vi "Main.vi"() -> ()   [LabVIEW 2015]
doc: "The myRIO Project template acquires acceleration data from the onboard accelerometer and displays the changes of acceleration values in a waveform chart."
uses:
  <vilib>/myRIO/Instrument Drivers/Onboard IO/PWM/typedefs/PWM Reference.ctl
  <vilib>/myRIO/Common/Instrument Driver Framework/Utilities/typedefs/myRIO Generic Hardware Reference.ctl
  <vilib>/myRIO/Common/Instrument Driver Framework/Utilities/typedefs/Hardware Version Enum.ctl
  <vilib>/myRIO/Common/Instrument Driver Framework/Utilities/typedefs/myRIO v1.0 Reference.ctl
  <vilib>/myRIO/Common/Instrument Driver Framework/Utilities/typedefs/Generic FPGA Reference.ctl
  <vilib>/myRIO/Common/Instrument Driver Framework/myRIO v1.0/PWM/typedefs/PWM Channels Enum.ctl
  <vilib>/myRIO/Instrument Drivers/Onboard IO/PWM/typedefs/PWM Configuration.ctl
  <vilib>/userdefined/High Color/nirio_resource_hc.ctl
  <vilib>/myRIO/Instrument Drivers/Onboard IO/DIO/typedefs/DIO Reference.ctl
  <vilib>/myRIO/Common/Instrument Driver Framework/myRIO v1.0/DIO/typedefs/DIO Channels List.ctl
  <vilib>/myRIO/Common/Instrument Driver Framework/myRIO v1.0/DIO/typedefs/DIO Channels Enum.ctl
  <vilib>/myRIO/Instrument Drivers/Onboard Devices/Accelerometer/typedefs/Accelerometer Reference.ctl
  <vilib>/myRIO/Common/Instrument Driver Framework/myRIO v1.0/Accelerometer/typedefs/Accelerometer Channels List.ctl
  <vilib>/myRIO/Common/Instrument Driver Framework/myRIO v1.0/Accelerometer/typedefs/Accelerometer Channels Enum.ctl
  <vilib>/myRIO/Common/Instrument Driver Framework/Utilities/vis/Is FPGA Ref Available.vi
  <vilib>/myRIO/Common/Instrument Driver Framework/myRIO v1.0/DIO/vis/myRIO v1.1 Open DIO.vi
  <vilib>/myRIO/Instrument Drivers/Onboard IO/DIO/vis/Read.vi
  <vilib>/myRIO/Instrument Drivers/Onboard IO/DIO/vis/Write.vi
  <vilib>/myRIO/Common/Instrument Driver Framework/myRIO v1.0/PWM/vis/myRIO v1.1 Open PWM.vi
  <vilib>/myRIO/Instrument Drivers/Onboard IO/PWM/vis/Set Duty Cycle and Frequency.vi
  <vilib>/myRIO/Common/Instrument Driver Framework/myRIO v1.0/Accelerometer/vis/myRIO v1.1 Open Accelerometer.vi
  <vilib>/myRIO/Instrument Drivers/Onboard Devices/Accelerometer/vis/Read.vi
  <vilib>/myRIO/Common/Instrument Driver Framework/Utilities/vis/Validate Channels.vi
  <vilib>/myRIO/Common/Instrument Driver Framework/myRIO v1.0/DIO/vis/myRIO v1.0 Reserve DIO.vi
  <vilib>/myRIO/Common/Instrument Driver Framework/myRIO v1.0/PWM/vis/myRIO v1.0 Reserve PWM.vi
  <vilib>/myRIO/Common/Instrument Driver Framework/myRIO v1.0/Accelerometer/vis/myRIO v1.0 Reserve Accelerometer.vi
  <vilib>/myRIO/Common/Instrument Driver Framework/myRIO v1.0/UART/vis/myRIO v1.0 Close UART.vi
  <vilib>/myRIO/Common/Instrument Driver Framework/myRIO v1.0/Resource Manager/vis/myRIO v1.0 Reserve Channel List.vi
  <vilib>/myRIO/Common/Instrument Driver Framework/myRIO v1.0/DIO/vis/myRIO v1.0 Build MUX Configuration DIO.vi
  <vilib>/myRIO/Common/Instrument Driver Framework/myRIO v1.0/PWM/vis/myRIO v1.0 Build MUX Configuration PWM.vi
  <vilib>/myRIO/Common/Instrument Driver Framework/myRIO v1.0/Accelerometer/vis/myRIO v1.0 Build MUX Configuration Accelerometer.vi
  <vilib>/myRIO/Common/Instrument Driver Framework/myRIO v1.0/Resource Manager/vis/myRIO v1.0 Reserve Channel.vi
  <vilib>/myRIO/Common/Instrument Driver Framework/myRIO v1.0/Resource Manager/vis/myRIO v1.0 Unreserve Channel.vi
  <vilib>/myRIO/Common/Instrument Driver Framework/myRIO v1.0/Resource Manager/vis/myRIO v1.0 Create Configuration List.vi
  <vilib>/myRIO/Common/Instrument Driver Framework/myRIO v1.0/Resource Manager/vis/myRIO v1.0 Build Mutex Name.vi
  <vilib>/Utility/VariantDataType/GetNumericInfo.vi
  <vilib>/Utility/error.llb/Error Cluster From Error Code.vi
  <vilib>/myRIO/Common/Instrument Driver Framework/myRIO v1.0/myRIO v1.1 Open.vi
  <vilib>/myRIO/Common/Instrument Driver Framework/Utilities/vis/IO Manager.vi
  <vilib>/myRIO/Common/Instrument Driver Framework/Utilities/vis/Configuration Manager.vi
  <vilib>/myRIO/Common/Instrument Driver Framework/myRIO v1.0/Resource Manager/vis/myRIO v1.0 Configure IO.vi
  <vilib>/myRIO/Common/Instrument Driver Framework/myRIO v1.0/myRIO v1.0 Close.vi
  <vilib>/myRIO/Common/Instrument Driver Framework/myRIO v1.0/DIO/vis/myRIO v1.0 Write DIO.vi
  <vilib>/myRIO/Common/Instrument Driver Framework/myRIO v1.0/PWM/vis/myRIO v1.0 Write PWM.vi
  <vilib>/myRIO/Common/Instrument Driver Framework/myRIO v1.0/DIO/vis/myRIO v1.0 Read DIO.vi
  <vilib>/myRIO/Common/Instrument Driver Framework/myRIO v1.0/Accelerometer/vis/myRIO v1.0 Get Scaling Constant Accelerometer.vi
  <vilib>/myRIO/Common/Instrument Driver Framework/myRIO v1.0/Accelerometer/vis/myRIO v1.0 Read Accelerometer.vi
  <vilib>/myRIO/Common/Instrument Driver Framework/Utilities/vis/FPGA Ref Manager.vi
  <vilib>/myRIO/Common/Instrument Driver Framework/myRIO v1.0/myRIO v1.0 Reset FPGA.vi
  <vilib>/myRIO/Common/Instrument Driver Framework/myRIO v1.0/IRQ/vis/myRIO v1.0 IRQ Info FGV.vi
  <vilib>/myRIO/Common/Instrument Driver Framework/myRIO v1.0/IRQ/vis/myRIO v1.0 Timer IRQ Info FGV.vi
  <vilib>/myRIO/Common/Instrument Driver Framework/myRIO v1.0/IRQ/vis/myRIO v1.0 ISR Agent.vi
  <vilib>/myRIO/Express VI/Onboard IO/DO/DO Express VI.xnode
  <vilib>/myRIO/Instrument Drivers/Onboard IO/DIO/vis/myRIO DIO Open.xnode
  <vilib>/myRIO/Express VI/Onboard IO/PWM/PWM Express VI.xnode
  <vilib>/myRIO/Instrument Drivers/Onboard IO/PWM/vis/myRIO PWM Open.xnode
  <vilib>/myRIO/Express VI/Onboard IO/DI/DI Express VI.xnode
  <vilib>/myRIO/Express VI/Onboard Devices/Accelerometer/Accelerometer Express VI.xnode
  <vilib>/myRIO/Instrument Drivers/Onboard Devices/Accelerometer/vis/myRIO Accelerometer Open.xnode
  <vilib>/myRIO/Instrument Drivers/Utilities/Utilities.lvlib
  <vilib>/myRIO/Instrument Drivers/Onboard Devices/Accelerometer/Accelerometer.lvlib
  <vilib>/myRIO/Instrument Drivers/Onboard IO/PWM/PWM.lvlib
  <vilib>/myRIO/Instrument Drivers/Onboard IO/DIO/DIO.lvlib
  <vilib>/ptbypt/NI_PtbyPt.lvlib
panel:
  out "结果":dbl
  out "X-Axis":dbl
  out "波形图表":T1(graph)
  out "error out":errorcluster
  # "Overview: The myRIO Project template acquires acceleration data from the onboard accelerometer and displays the changes of acceleration values in a waveform chart.\nInstructions:\n1. Check the myRIO target IP address in the project and make sure the target IP address is correct. \n2. Run this VI."
  # "左 29"
  # "右31"
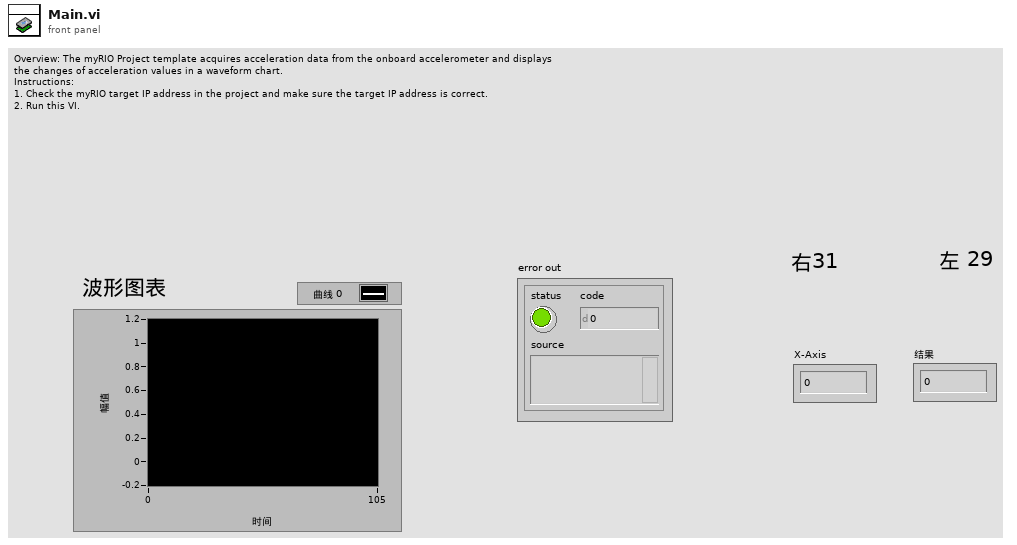
[diagram p1: front panel]
types:
  T1 = cluster{"X-Axis":dbl, "Y-Axis":dbl, "Z-Axis":dbl}
  T2 = typedef "PWM.lvlib/PWM Reference.ctl" = cluster{"myRIO Reference":T3, "PWM Channels Enum":T7, "PWM Configuration":T8}
  T3 = typedef "myRIO Generic Hardware Reference.ctl" = cluster{"myRIO Model":T4, "myRIO Hardware Reference":T5}
  T4 = typedef "Hardware Version Enum.ctl" = enum16{"Unknown", "myRIO-1900", "myRIO-1950", "roboRIO"}
  T5 = typedef "myRIO v1.0 Reference.ctl" = cluster{"Generic FPGA Reference":T6, "Allow multiple opens":bool}
  T6 = typedef "Generic FPGA Reference.ctl" = refnum<k20>
  T7 = typedef "PWM Channels Enum.ctl" = enum16{"Not Connected", "C/PWM0", "C/PWM1", "A/PWM0", "A/PWM1", "A/PWM2", "B/PWM0", "B/PWM1", "B/PWM2", "PWM/PWM0", "PWM/PWM1", "PWM/PWM2", "PWM/PWM3", "PWM/PWM4", "PWM/PWM5", "PWM/PWM6", "PWM/PWM7", "PWM/PWM8", "PWM/PWM9"}
  T8 = typedef "PWM.lvlib/PWM Configuration.ctl" = cluster{"Frequency":dbl, "Duty Cycle":dbl}
  T9 = typedef "nirio_resource_hc.ctl" = tag
  T10 = typedef "DIO.lvlib/DIO Reference.ctl" = cluster{"myRIO Reference":T3, "DIO Channels List":T11}
  T11 = typedef "DIO Channels List.ctl" = T12[]
  T12 = typedef "DIO Channels Enum.ctl" = enum16{"Not Connected", "C/DIO0", "C/DIO1", "C/DIO2", "C/DIO3", "C/DIO4", "C/DIO5", "C/DIO6", "C/DIO7", "A/DIO0", "A/DIO1", "A/DIO2", "A/DIO3", "A/DIO4", "A/DIO5", "A/DIO6", "A/DIO7", "A/DIO8", "A/DIO9", "A/DIO10", "A/DIO11", "A/DIO12", "A/DIO13", "A/DIO14", "A/DIO15", "B/DIO0", "B/DIO1", "B/DIO2", "B/DIO3", "B/DIO4", "B/DIO5", "B/DIO6", "B/DIO7", "B/DIO8", "B/DIO9", "B/DIO10", "B/DIO11", "B/DIO12", "B/DIO13", "B/DIO14", "B/DIO15", "LED0", "LED1", "LED2", "LED3", "Button0", "DIO/DIO0", "DIO/DIO1", "DIO/DIO2", "DIO/DIO3", "DIO/DIO4", "DIO/DIO5", "DIO/DIO6", "DIO/DIO7", "DIO/DIO8", "DIO/DIO9", "SPI/CS0", "SPI/CS1", "SPI/CS2", "SPI/CS3", "LED RADIO (Green)", "LED RADIO (Red)", "LED COMM (Green)", "LED COMM (Red)", "LED MODE (Green)", "LED MODE (Red)"}
  T13 = typedef "Accelerometer.lvlib/Accelerometer Reference.ctl" = cluster{"myRIO Reference":T3, "Accelerometer Channels List":T14, "LSB Weight":dbl}
  T14 = typedef "Accelerometer Channels List.ctl" = T15[]
  T15 = typedef "Accelerometer Channels Enum.ctl" = enum16{"Not Connected", "X-Axis", "Y-Axis", "Z-Axis"}
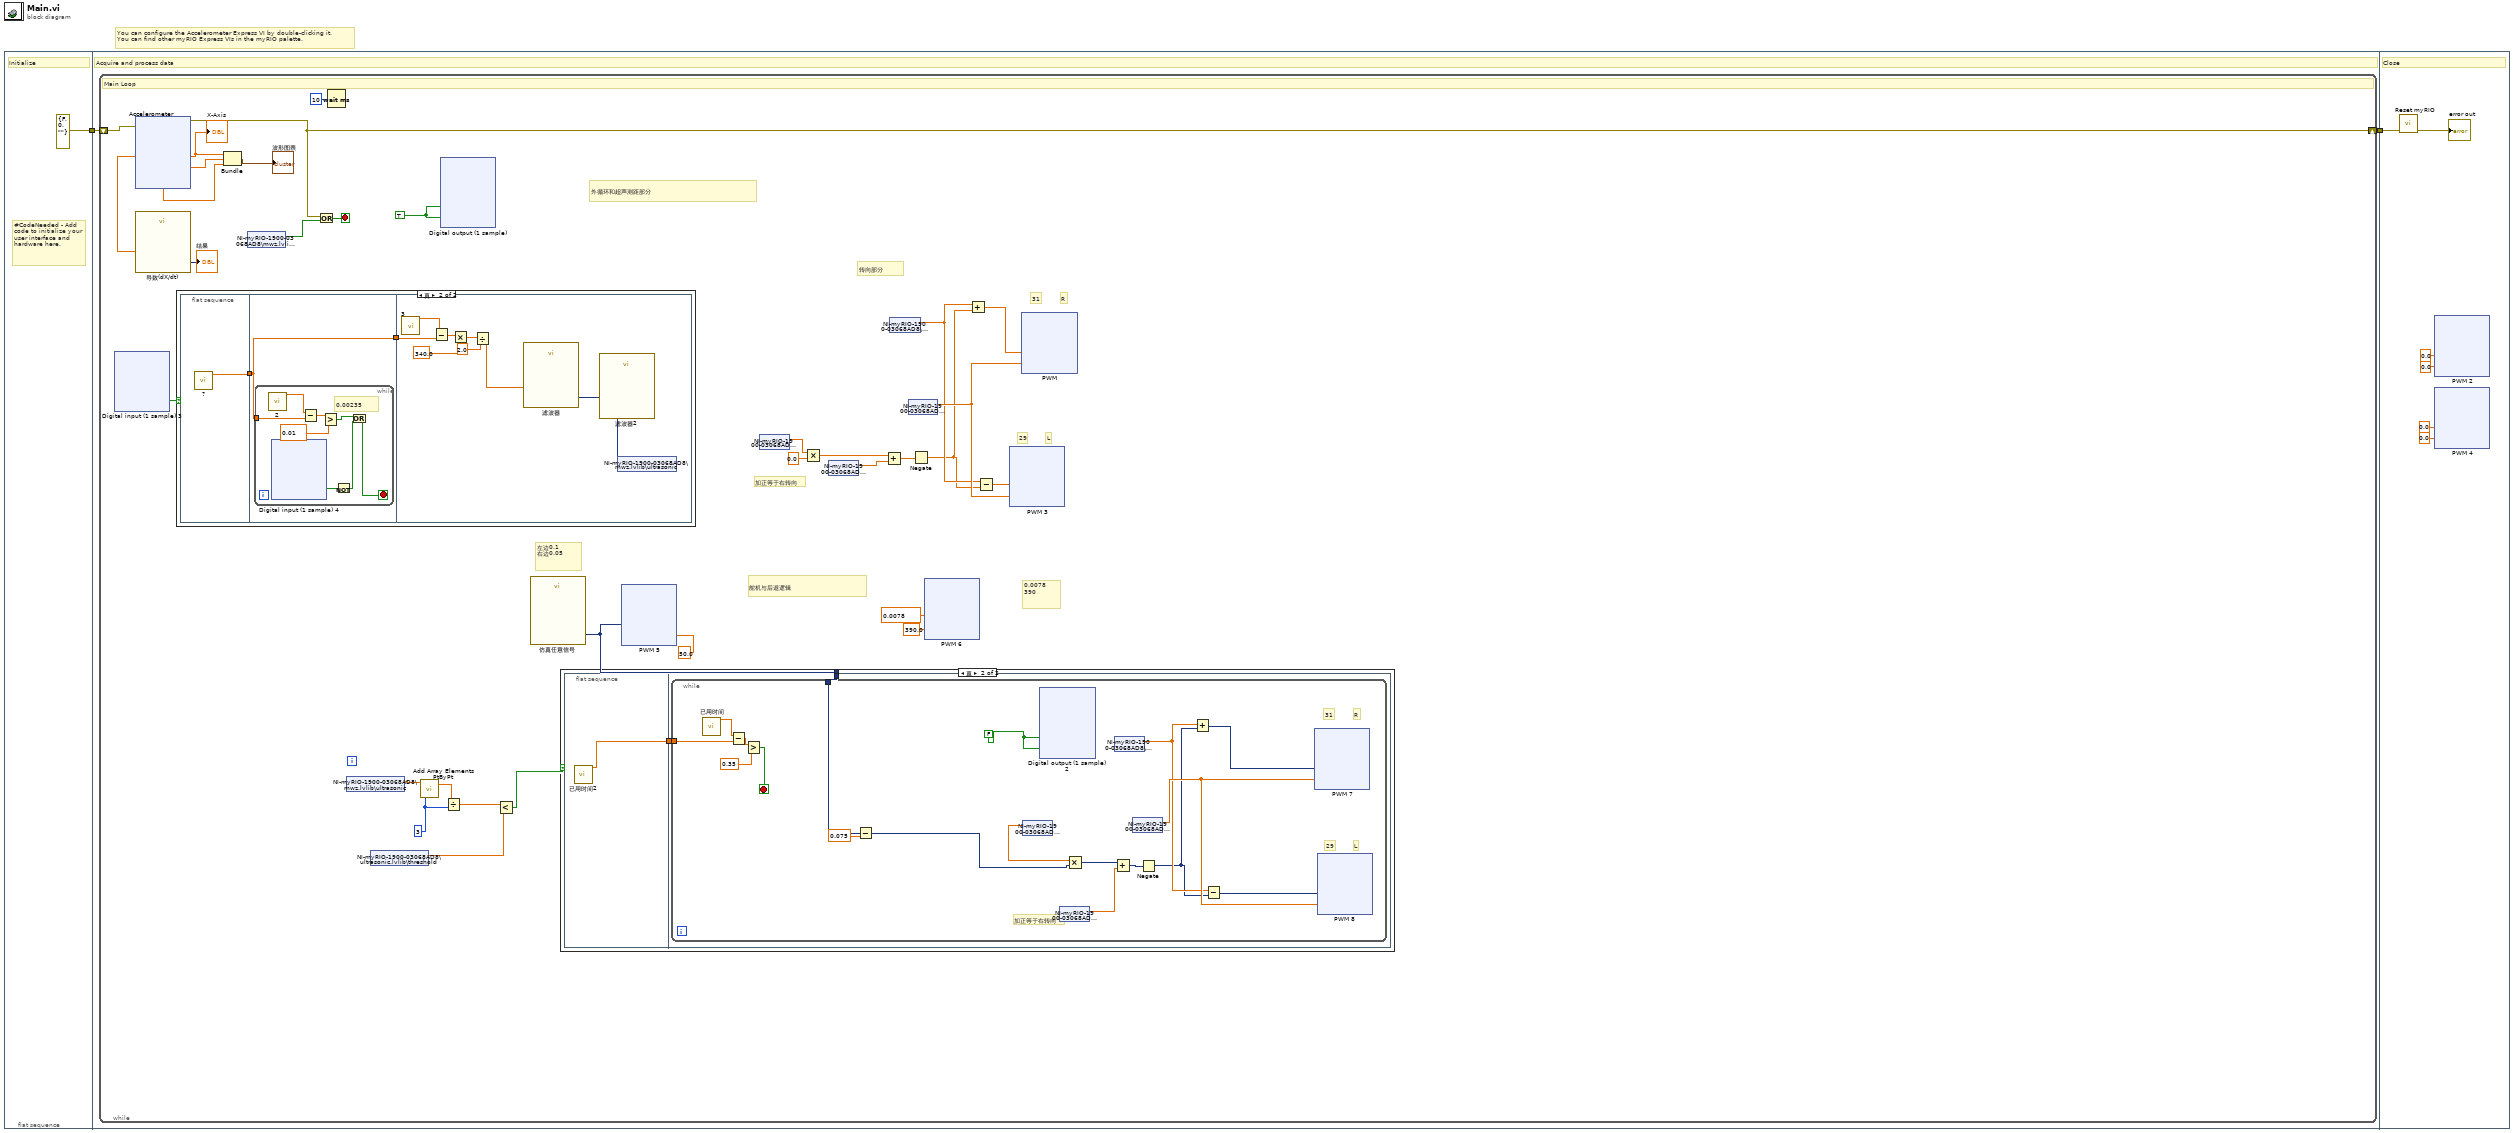
[diagram p0: block diagram]
diagram:
  # "You can configure the Accelerometer Express VI by double-clicking it.\nYou can find other myRIO Express VIs in the myRIO palette."
  n1 = flat-sequence {
    tunnel: [errorcluster {"status"=FALSE, "code"=0, "source"=""} ("error in (no error)")] -> w2
    tunnel: w2 -> [w5]
    tunnel: [w4] -> w1
    tunnel: w1 -> [w478]
    frame #0 {
      # "#CodeNeeded - Add code to initialize your user interface and hardware here."
      # "Initialize"
    }
    frame #1 {
      # "Acquire and process data"
      n2 = while {
        shift-right: [w35] -> w4
        shift-left: w5 -> [w25]
        stop <- w37 stop-if-true
        w7 = 3 ("sample length")
        w11 = TRUE
        # "舵机与后退逻辑"
        # "转向部分"
        # "外循环和超声测距部分"
        # "0.0078\n390"
        # "左边0.1\n右边0.05"
        # "L"
        # "R"
        # "加正等于右转向"
        # "29"
        # "31"
        # "Main Loop"
        n3 = xnode "Digital input (1 sample) 3"() -> ("B/DIO15 (Pin 34)"=w22:bool)  [unwired: 1 in, 1 out]
        n4 = xnode "Accelerometer"("error in (no error)"=w25) -> ("X-Axis"=w24:dbl, "Y-Axis"=w34:dbl, "Z-Axis"=w33:dbl, "error out"=w35:errorcluster)
        "X-Axis" <- w24
        n5 = call "导数(dX/dt)"("Signals"=w24) -> ("Result"=→"结果":dynamicdata)  [unwired: 5 in, 1 out]
        n6 = case shown="真" w22 {
          frame False {
          }
          frame True {
            n7 = flat-sequence {
              tunnel: [w204] -> w203
              tunnel: w203 -> [w205]
              tunnel: [w205] -> w202
              tunnel: w202 -> [w256]
              frame #0 {
                n8 = call "?"() -> ("Present (s)"=w204:dbl)  [unwired: 12 in, 7 out]
              }
              frame #1 {
                n9 = while {
                  tunnel: w205 -> [w212]
                  stop <- w206 stop-if-true
                  # "0.00235"
                  n10 = call "2"() -> ("Present (s)"=w213:dbl)  [unwired: 12 in, 7 out]
                  n11 = xnode "Digital input (1 sample) 4"() -> ("B/DIO15 (Pin 34)"=w208:bool)  [unwired: 1 in, 1 out]
                  n12 = Subtract(x=w213, y=w212) -> (x-y=w211:dbl)
                  n13 = Greater?(x=w211, y=0.01) -> (0:w209:bool)
                  n14 = Not(x=w208) -> (.not. x?=w207:bool)
                  n15 = Or(x=w209, y=w207) -> (x .or. y?=w206:bool)
                }
              }
              frame #2 {
                n16 = call "3"() -> ("Present (s)"=w257:dbl)  [unwired: 12 in, 7 out]
                n17 = Subtract(x=w257, y=w256) -> (x-y=w255:dbl)
                n18 = Multiply(x=w255, y=340.0) -> (x*y=w253:dbl)
                n19 = Divide(x=w253, y=2.0) -> (x/y=w251:dbl)
                n20 = call "滤波器"("Signal"=w251) -> ("Filtered Signal"=w250:dynamicdata)  [unwired: 9 in, 1 out]
                n21 = call "滤波器2"("Signal"=w250) -> ("Filtered Signal"=w249:dynamicdata)  [unwired: 9 in, 1 out]
                n22 = shared-variable "NI-myRIO-1900-03068AD8\\mwz.lvlib\\ultrasonic"(w249) -> ()  [unwired: 1 in, 1 out]
              }
            }
          }
        }
        n23 = Bundle("X-Axis"=w24, "Y-Axis"=w34, "Z-Axis"=w33) -> (→"波形图表":T1)  [unwired: 1 in]
        n24 = shared-variable "NI-myRIO-1900-03068AD8\\mwz.lvlib\\OFF"() -> (w31:bool)  [unwired: 1 in, 1 out]
        n25 = Or(x=w35, y=w31) -> (x .or. y?=w37:bool)
        n26 = Wait (ms)(milliseconds to wait=u32 10) -> ()  [unwired: 1 out]
        n27 = shared-variable "NI-myRIO-1900-03068AD8\\mwz.lvlib\\ultrasonic"() -> (w9:dbl)  [unwired: 1 in, 1 out]
        n28 = shared-variable "NI-myRIO-1900-03068AD8\\ultrasonic.lvlib\\threshold"() -> (w10:dbl)  [unwired: 1 in, 1 out]
        n29 = call <vilib>:"Add Array Elements PtByPt.vi"("sample length"=w7, "input data point"=w9) -> ("sum"=w8:dbl)  [unwired: 2 in, 1 out]
        n30 = xnode "Digital output (1 sample)"("L (C/DIO0 (DIO0))"=w11, "R (C/DIO1 (DIO1))"=w11) -> ()  [unwired: 1 in, 1 out]
        n31 = Divide(x=w8, y=w7) -> (x/y=w6:dbl)
        n32 = Less?(x=w6, y=w10) -> (x < y?=w16:bool)
        n33 = call "仿真任意信号"() -> ("Signal"=w15:dynamicdata)  [unwired: 9 in, 2 out]
        n34 = case shown="真" w16 {
          tunnel: w15 -> [_ w39]
          frame False {
          }
          frame True {
            n35 = flat-sequence {
              tunnel: [w40] -> w38
              tunnel: w39 -> [w41]
              tunnel: w38 -> [w42]
              frame #0 {
                n36 = call "已用时间2"() -> ("Present (s)"=w40:dbl)  [unwired: 12 in, 7 out]
              }
              frame #1 {
                n37 = while {
                  tunnel: w42 -> [w57]
                  tunnel: w41 -> [w45]
                  stop <- w60 stop-if-true
                  w43 = FALSE ("L (C/DIO0 (DIO0))")
                  # "L"
                  # "R"
                  # "加正等于右转向"
                  # "29"
                  # "31"
                  n38 = call "已用时间"() -> ("Present (s)"=w58:dbl)  [unwired: 12 in, 7 out]
                  n39 = Subtract(x=w58, y=w57) -> (x-y=w56:dbl)
                  n40 = Greater?(x=w56, y=0.35) -> (0:w60:bool)
                  n41 = Subtract(x=w45, y=0.075) -> (x-y=w46:dynamicdata)
                  n42 = shared-variable "NI-myRIO-1900-03068AD8\\ultrasonic.lvlib\\x"() -> (w47:dbl)  [unwired: 1 in, 1 out]
                  n43 = xnode "Digital output (1 sample) 2"("L (C/DIO0 (DIO0))"=w43, "R (C/DIO1 (DIO1))"=w43) -> ()  [unwired: 1 in, 1 out]
                  n44 = shared-variable "NI-myRIO-1900-03068AD8\\mwz.lvlib\\L"() -> (w49:dbl)  [unwired: 1 in, 1 out]
                  n45 = Multiply(x=w47, y=w46) -> (x*y=w48:dynamicdata)
                  n46 = shared-variable "NI-myRIO-1900-03068AD8\\mwz.lvlib\\R"() -> (w52:dbl)  [unwired: 1 in, 1 out]
                  n47 = Add(x=w48, y=w49) -> (x+y=w50:dynamicdata)
                  n48 = shared-variable "NI-myRIO-1900-03068AD8\\mwz.lvlib\\F"() -> (w55:dbl)  [unwired: 1 in, 1 out]
                  n49 = Negate(x=w50) -> (-x=w51:dynamicdata)
                  n50 = Add(x=w52, y=w51) -> (x+y=w53:dynamicdata)
                  n51 = Subtract(x=w52, y=w51) -> (x-y=w54:dynamicdata)
                  n52 = xnode "PWM 7"("Duty Cycle"=w53, "Frequency [Hz]"=w55) -> ()  [unwired: 1 in, 1 out]
                  n53 = xnode "PWM 8"("Duty Cycle"=w54, "Frequency [Hz]"=w55) -> ()  [unwired: 1 in, 1 out]
                }
              }
            }
          }
        }
        n54 = xnode "PWM 5"("Duty Cycle"=w15, "Frequency [Hz]"=50.0) -> ()  [unwired: 1 in, 1 out]
        n55 = shared-variable "NI-myRIO-1900-03068AD8\\ultrasonic.lvlib\\x"() -> (w17:dbl)  [unwired: 1 in, 1 out]
        n56 = Multiply(x=w17, y=0.0) -> (x*y=w18:dbl)
        n57 = shared-variable "NI-myRIO-1900-03068AD8\\mwz.lvlib\\L"() -> (w19:dbl)  [unwired: 1 in, 1 out]
        n58 = Add(x=w18, y=w19) -> (x+y=w20:dbl)
        n59 = shared-variable "NI-myRIO-1900-03068AD8\\mwz.lvlib\\R"() -> (w27:dbl)  [unwired: 1 in, 1 out]
        n60 = shared-variable "NI-myRIO-1900-03068AD8\\mwz.lvlib\\F"() -> (w30:dbl)  [unwired: 1 in, 1 out]
        n61 = Negate(x=w20) -> (-x=w26:dbl)
        n62 = xnode "PWM 6"("Duty Cycle"=0.0078, "Frequency [Hz]"=390.0) -> ()  [unwired: 1 in, 1 out]
        n63 = Add(x=w27, y=w26) -> (x+y=w28:dbl)
        n64 = Subtract(x=w27, y=w26) -> (x-y=w29:dbl)
        n65 = xnode "PWM 3"("Duty Cycle"=w29, "Frequency [Hz]"=w30) -> ()  [unwired: 1 in, 1 out]
        n66 = xnode "PWM"("Duty Cycle"=w28, "Frequency [Hz]"=w30) -> ()  [unwired: 1 in, 1 out]
      }
    }
    frame #2 {
      # "Close"
      n67 = call <vilib>:"Reset myRIO.vi"("error in (no error)"=w478) -> ("error out"=→"error out":errorcluster)  [unwired: 10 in]
      n68 = xnode "PWM 2"("Duty Cycle"=0.0, "Frequency [Hz]"=0.0) -> ()  [unwired: 1 in, 1 out]
      n69 = xnode "PWM 4"("Duty Cycle"=0.0, "Frequency [Hz]"=0.0) -> ()  [unwired: 1 in, 1 out]
    }
  }
